vi "simpleRobotController.vi"() -> ()   [LabVIEW 2012]
panel:
  in  "Control Panel":T1(tab)
  in  "Steering Angle":dbl(knob) scale=0.0..360.0
  out "Heading":dbl(knob) scale=0.0..360.0
  out "Commanded Steering Angle":dbl(graph)
  in  "Steering Angle Debug":dbl(knob) scale=0.0..360.0
  in  "Desired Heading":dbl(slide) scale=0.0..360.0
  out "Heading Chart":cluster{"Desired Heading":dbl, dbl}(graph)
  in  "estop":bool
  out "Robot Running":bool
  # "Click the arrow above to run this thing!"
  # "Derek Redfern\nProject 1"
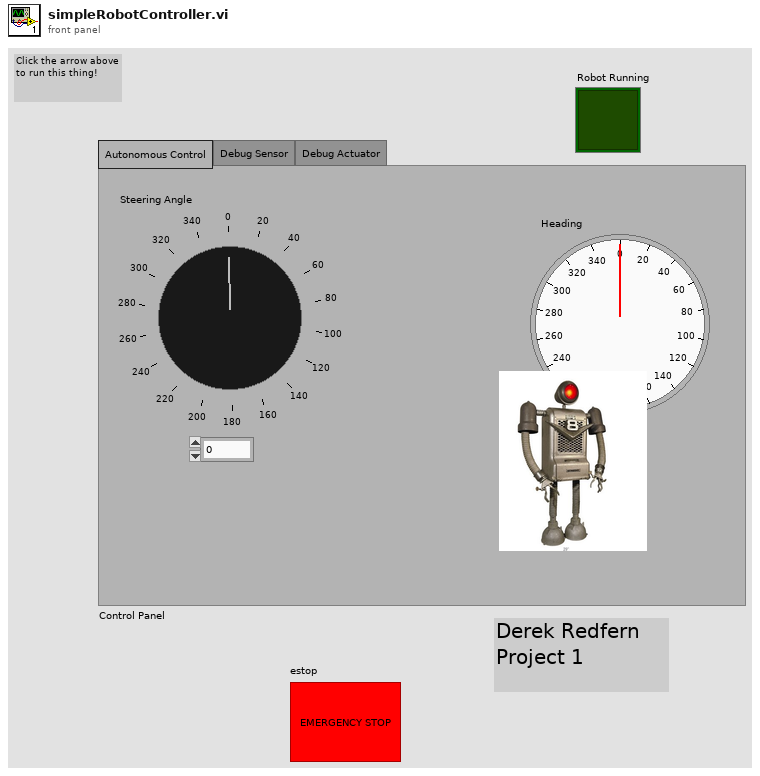
[diagram p1: front panel]
types:
  T1 = enum32{"Autonomous Control", "Debug Sensor", "Debug Actuator"}
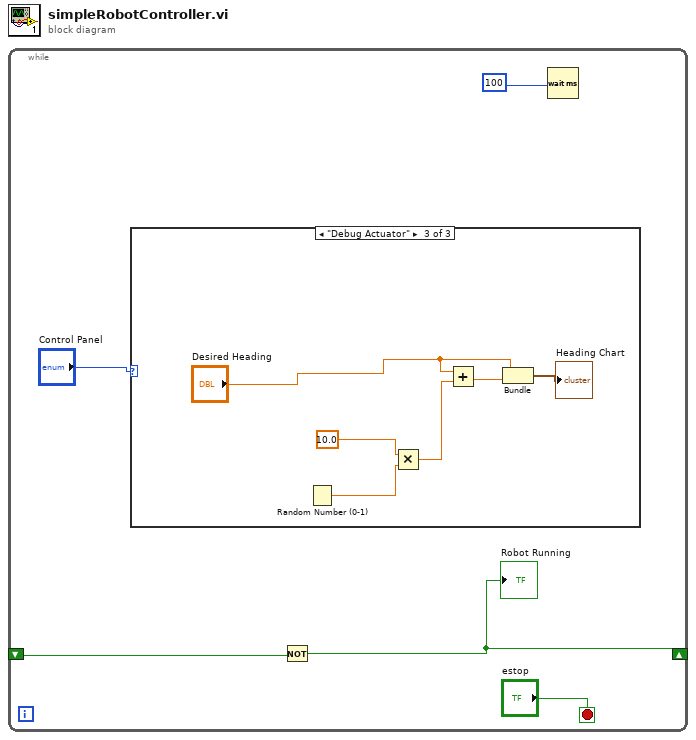
[diagram p0: block diagram]
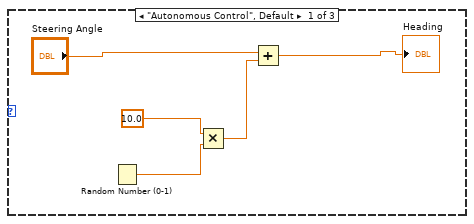
[diagram p2: hidden frame]
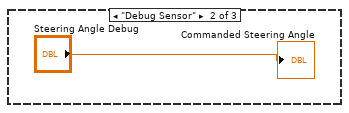
[diagram p3: hidden frame]
diagram:
  n1 = while {
    shift-right: [w4] -> _
    shift-left: _ -> [w3]
    stop <- "estop" stop-if-true
    n2 = case shown="\"Debug Actuator\"" "Control Panel" {
      frame "Autonomous Control", Default {
        n3 = Random Number (0-1)() -> (number: 0 to 1=w9:dbl)
        n4 = Multiply(x=10.0, y=w9) -> (x*y=w8:dbl)
        n5 = Add(x="Steering Angle", y=w8) -> (x+y=→"Heading":dbl)
      }
      frame "Debug Sensor" {
        "Commanded Steering Angle" <- "Steering Angle Debug"
      }
      frame "Debug Actuator" {
        n6 = Random Number (0-1)() -> (number: 0 to 1=w16:dbl)
        n7 = Multiply(x=10.0, y=w16) -> (x*y=w15:dbl)
        n8 = Add(x="Desired Heading", y=w15) -> (x+y=w13:dbl)
        n9 = Bundle("Desired Heading"="Desired Heading", w13) -> (→"Heading Chart":cluster{"Desired Heading":dbl, dbl})  [unwired: 1 in]
      }
    }
    n10 = Not(x=w3) -> (.not. x?=w4:bool)
    "Robot Running" <- w4
    n11 = Wait (ms)(milliseconds to wait=u32 100) -> ()  [unwired: 1 out]
  }
